vi "Dequeue.vi"(8 "error in (no error)":errorcluster, 11 "Transporter in":refnum<class "Transporter.lvclass">) -> (0 "error out":errorcluster, 2 "Abstract":refnum<class "Abstract.lvclass">)   [LabVIEW 2021, in "Msn Trasnsportation Library 1.lvlib" / "Transporter.lvclass"]
uses:
  Transporter.lvclass
  Abstract/Abstract.lvclass
  Transporter.lvclass/Transporter.ctl
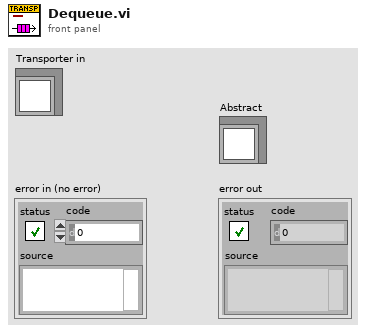
[diagram p1: front panel]
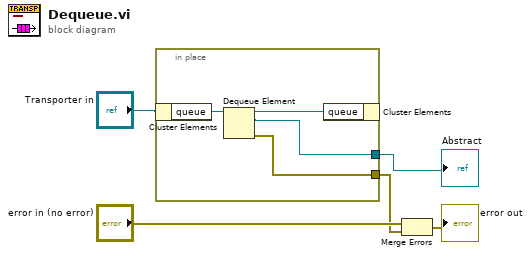
[diagram p0: block diagram]
diagram:
  n1 = in-place {
    in-place-border: [w7] -> w2
    in-place-border: [w6] -> w1
    n2 = in-place-cluster #1("Transporter in") -> ("queue"=w9:refnum<queue>)
    n3 = Dequeue Element(queue=w9) -> (queue out=w8:refnum<queue>, element=w6:refnum<class "Abstract.lvclass">, error out=w7:errorcluster)  [unwired: 2 in, 1 out]
    n4 = in-place-cluster #1("queue"=w8) -> ()  [unwired: 1 out]
  }
  "Abstract" <- w1
  n5 = Merge Errors("error in (no error)", w2) -> (→"error out":errorcluster)
